vi "Parse Charact Type.vi"(0 "Config File in":path, 11 "error in (no error)":errorcluster) -> (4 "Config File out":path, 6 "Charact type (scalar or vector)":string, 15 "error out":errorcluster)   [LabVIEW 2023, in "RFFixtureCharact.Public.lvlib"]
uses:
  RFFixtureCharact.Public.lvlib
  <vilib>/regexp/Match Regular Expression.xnode
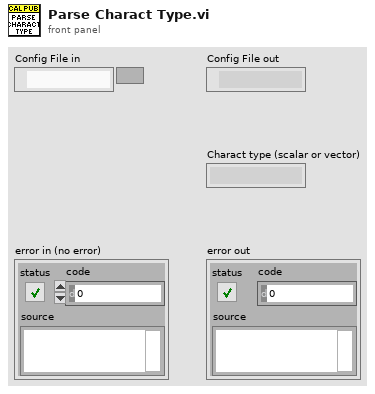
[diagram p1: front panel]
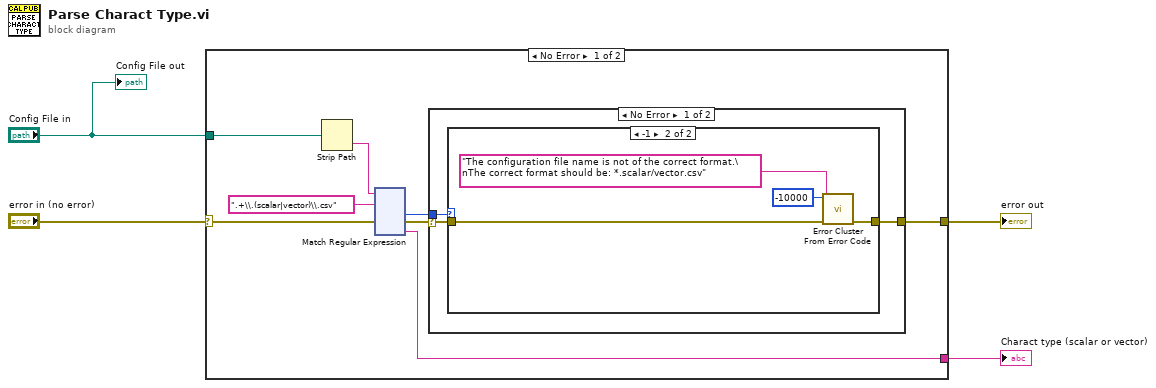
[diagram p0: block diagram]
diagram:
  n1 = case shown="No Error" "error in (no error)" {
    selector: "error in (no error)" -> [w10 w141]
    tunnel: [w5 _] -> w4
    tunnel: "Config File in" -> [w9 _]
    tunnel: [w6 w141] -> w1
    frame No Error {
      n2 = Strip Path(path=w9) -> (name=w12:string)  [unwired: 1 out]
      n3 = xnode "Match Regular Expression"("input string"=w12, "regular expression"=".+\\.(scalar|vector)\\.csv", "error in"=w10) -> ("offset past match"=w8:i32, "error out"=w7:errorcluster, "submatch 1"=w5:string)  [unwired: 3 in, 3 out]
      n4 = case shown="No Error" w7 {
        selector: w7 -> [w14 w21]
        tunnel: w8 -> [w15 _]
        tunnel: [w13 w21] -> w6
        frame No Error {
          n5 = case shown="-1" w15 {
            tunnel: w14 -> [w16 w20]
            tunnel: [w16 w19] -> w13
            frame Default {
            }
            frame -1 {
              n6 = call <vilib>:"Error Cluster From Error Code.vi"("error in (no error)"=w20, "error message (\"\")"="The configuration file name is not of the correct format.\nThe correct format should be: *.scalar/vector.csv" ("error message (\"\")"), "error code (0)"=-10000) -> ("error out"=w19:errorcluster)  [unwired: 6 in]
            }
          }
        }
        frame Error {
        }
      }
    }
    frame Error {
    }
  }
  "error out" <- w1
  "Charact type (scalar or vector)" <- w4
  "Config File out" <- "Config File in"
